vi "Get Events.vi"(11 "Create Project View in":refnum<class "Edit Project View.lvclass">) -> (2 "Events":T1, 3 "Create Project View out":refnum<class "Edit Project View.lvclass">)   [LabVIEW 2013, in "Edit Project View.lvlib" / "Edit Project View.lvclass"]
uses:
  Edit Project View.lvclass
  Typedef/Events.ctl
  Edit Project View.lvclass/Edit Project View.ctl
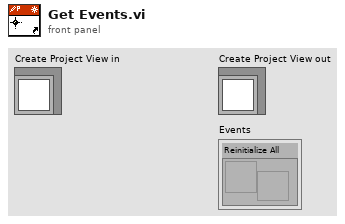
[diagram p1: front panel]
types:
  T1 = typedef "Edit Project View.lvlib/Edit Project View.lvclass/Events.ctl" = cluster{"Reinitialize All":refnum<user-event>}
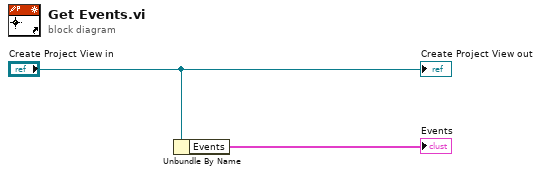
[diagram p0: block diagram]
diagram:
  n1 = Unbundle By Name("Create Project View in") -> ("Events"=→"Events":T1)
  "Create Project View out" <- "Create Project View in"
